vi "lvEtherbone.device_flush.vi"(0 "eb_socket_ID":i32, 1 "eb_device_ID":i32, 5 "error in (no error)":errorcluster) -> (14 "eb_socket_ID out":i32, 15 "eb_device_ID out":i32, 19 "error out":errorcluster)   [LabVIEW 2009, in "lvEtherbone.lvlib"]
doc: "//-----------------------------------------------------------------------------------\n// author : Dietrich Beck, GSI-Darmstadt\n// purpose : Flush commands queued on the device out the socket.\n// returns : lveb_status_t\n//-----------------------------------------------------------------------------------\nETHERBONE_API int lveb_device_flush(int eb_deviceID //ID of Wishbone device\n );"
uses:
  lvEtherbone.lvlib
  bin/lvEtherbone.dll
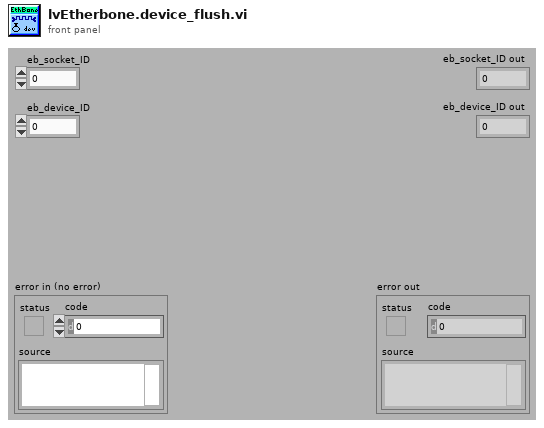
[diagram p1: front panel]
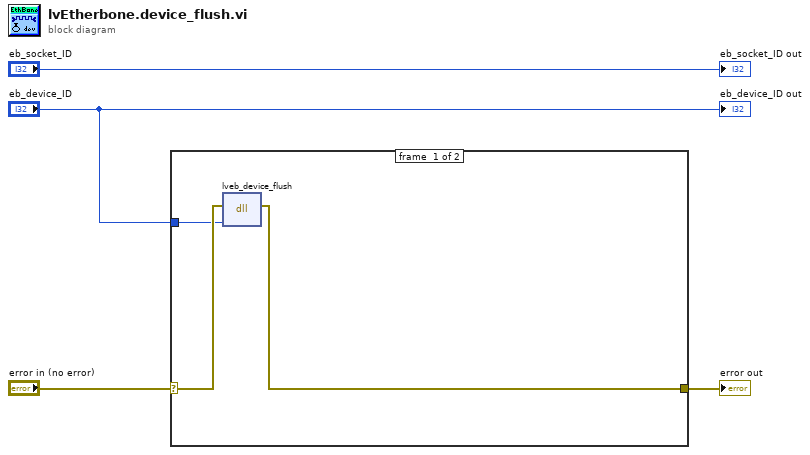
[diagram p0: block diagram]
diagram:
  n1 = case shown="No Error" "error in (no error)" {
    selector: "error in (no error)" -> [w7 w8]
    tunnel: [w5 w8] -> w3
    tunnel: "eb_device_ID" -> [w6 _]
    frame #0 {
      n2 = dll-call lib="F:/beck/Project/BEL/SCC/etherbone-core/api/lvEtherbone/bin/lvEtherbone.*" fn="lveb_device_flush"(error in=w7, "eb_device_ID"=w6) -> (error out=w5:errorcluster)  [unwired: 4 in, 1 out]
    }
    frame #1 {
    }
  }
  "error out" <- w3
  "eb_socket_ID out" <- "eb_socket_ID"
  "eb_device_ID out" <- "eb_device_ID"
